vi "Main.vi"() -> ()   [LabVIEW 2026]
doc: "This LabVIEW application simulates scheduled programmatic heating and cooling control for heating, ventilation and air-conditioning (HVAC) system."
uses:
  controls/UI Data.ctl
  support/Message Queue/Enqueue Message (Single).vi
  <vilib>/Utility/error.llb/Error Cluster From Error Code.vi
  <vilib>/ErrorRing/Error Ring.xnode
  support/Message Queue/Message Queue.lvlib
  support/User Event - Stop/User Event - Stop.lvlib
  controls/Manual Override.ctl
  controls/System Status Displays.ctl
  controls/User Settings.ctl
panel:
  in  "User Settings":T1
  in  "Manual Override":T2
  out "System Status Displays":T3
  in  "Exit":bool
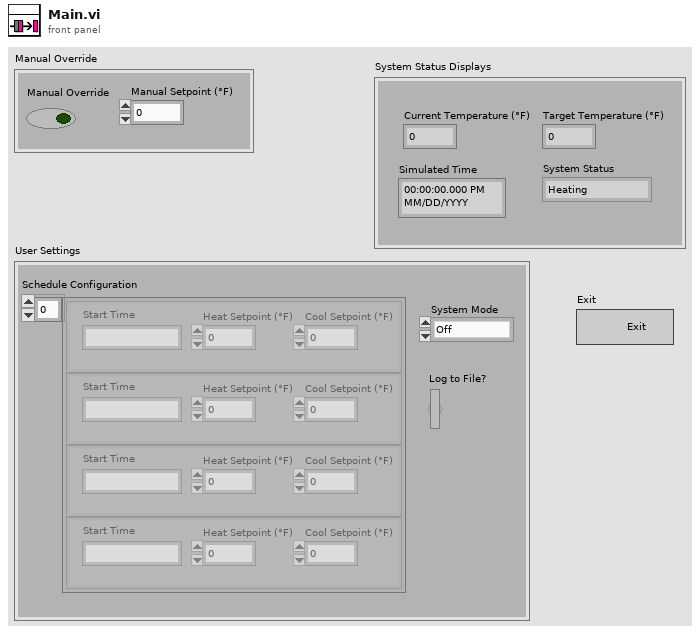
[diagram p1: front panel]
types:
  T1 = typedef "User Settings.ctl" = cluster{"Schedule Configuration":cluster{"Start Time":string, "Heat Setpoint (°F)":dbl, "Cool Setpoint (°F)":dbl}[], "System Mode":enum16{"Off", "Cool", "Auto", "Heat"}, "Log to File?":bool}
  T2 = typedef "Manual Override.ctl" = cluster{"Manual Override":bool, "Manual Setpoint (°F)":dbl}
  T3 = typedef "System Status Displays.ctl" = cluster{"Current Temperature (°F)":dbl, "Target Temperature (°F)":dbl, "System Status":enum16{"Heating", "Cooling", "Idle"}, "Simulated Time ":timestamp}
  T4 = typedef "UI Data.ctl" = cluster{"Boolean <Replace Me>":bool, "String <Replace Me>":string, "Numeric <Replace Me>":dbl, "Do Something Ref":refnum<vi>, "Do Something Else Ref":refnum<vi>, "Data Display Ref":refnum<vi>, "Exit Button Ref":refnum<vi>}
  T5 = typedef "Message Queue.lvlib/All Message Queues.ctl" = cluster{"UI":refnum<queue>}
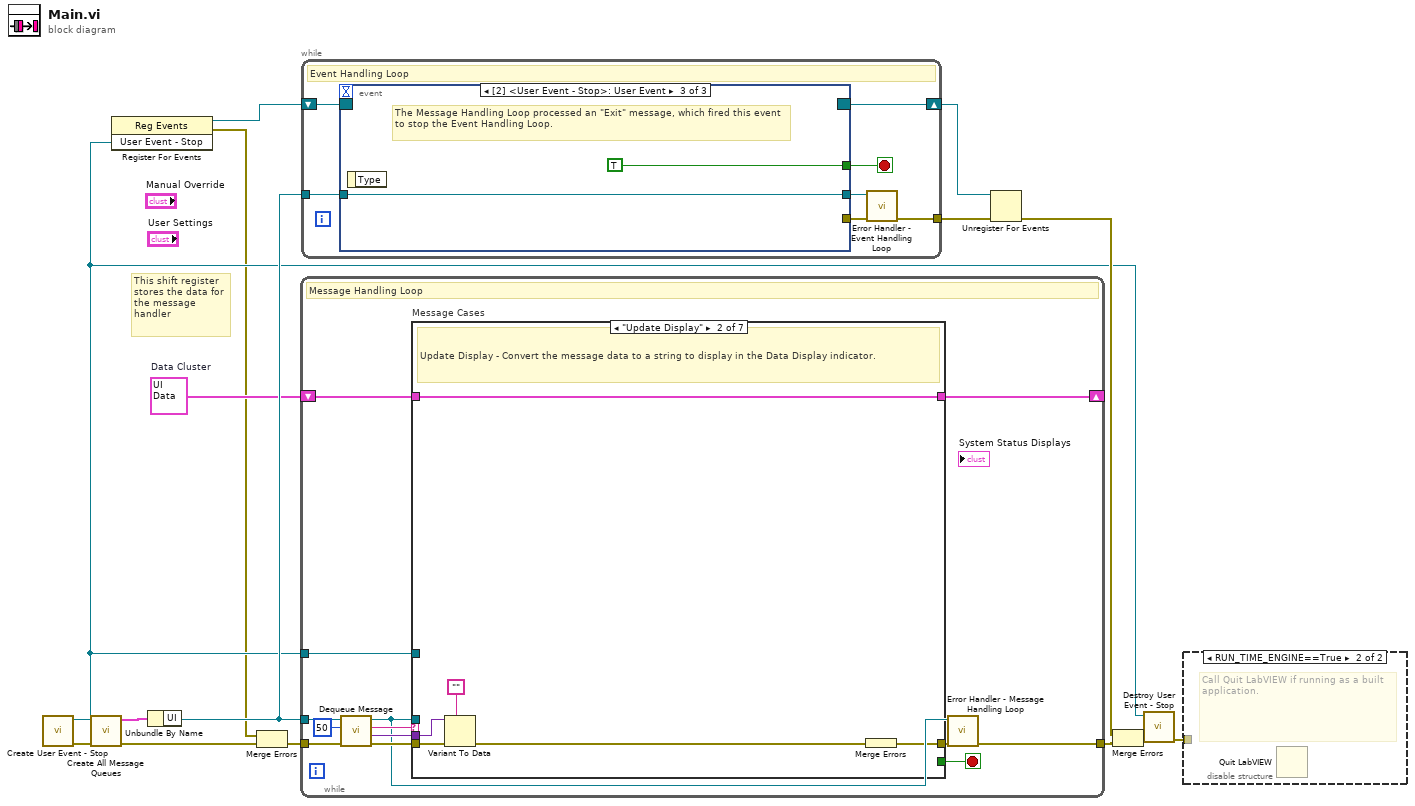
[diagram p0: block diagram]
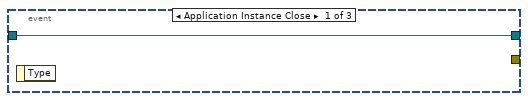
[diagram p3: hidden frame]
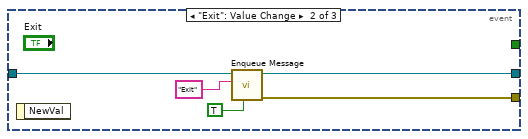
[diagram p4: hidden frame]
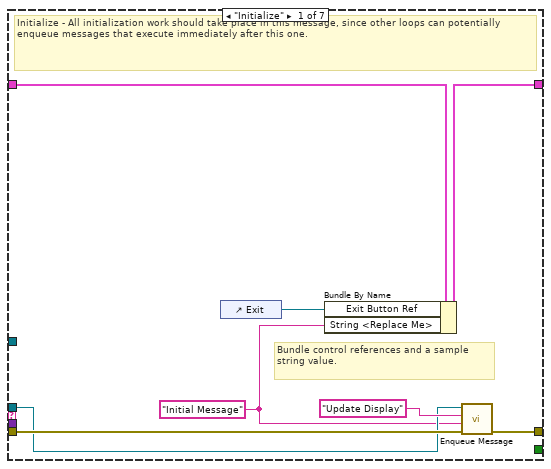
[diagram p5: hidden frame]
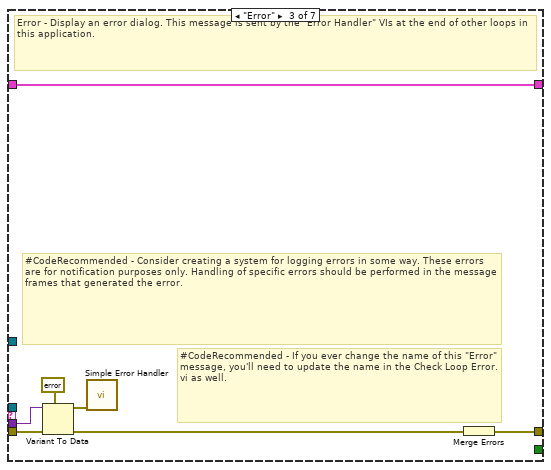
[diagram p6: hidden frame]
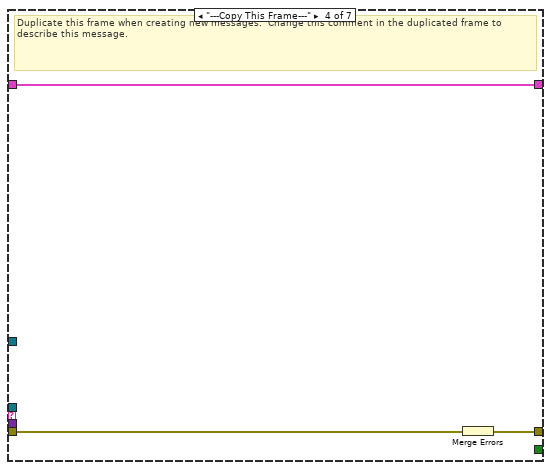
[diagram p7: hidden frame]
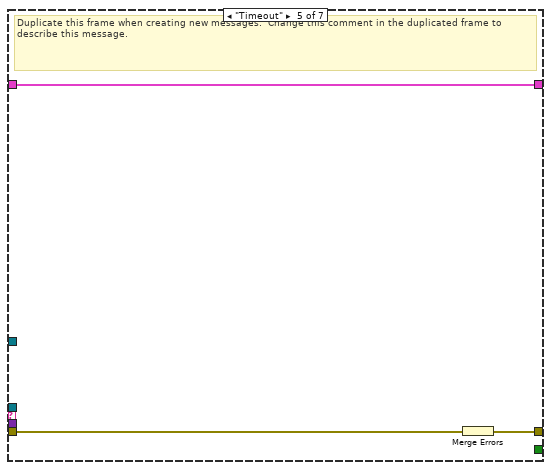
[diagram p8: hidden frame]
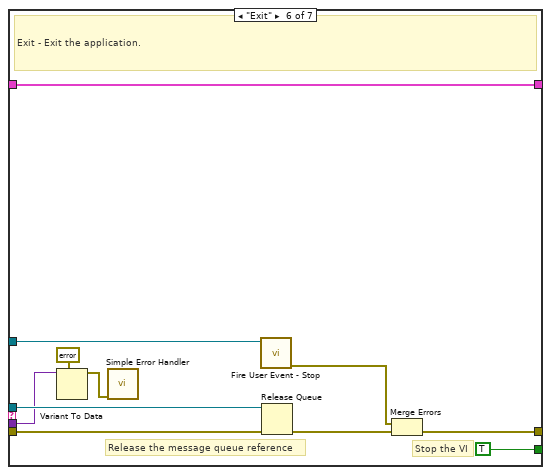
[diagram p9: hidden frame]
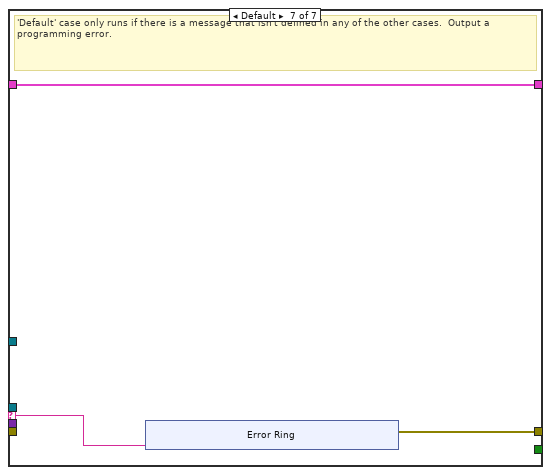
[diagram p10: hidden frame]
diagram:
  w7 = T4 {"Boolean <Replace Me>"=FALSE, "String <Replace Me>"="", "Numeric <Replace Me>"=0.0, "Do Something Ref"=refnum, "Do Something Else Ref"=refnum, "Data Display Ref"=refnum, "Exit Button Ref"=refnum}  # Data Cluster
  # "This shift register stores the data for the message handler"
  n1 = call "Create User Event - Stop.vi"() -> ("error out"=w11:errorcluster, "User Event - Stop"=w3:refnum<user-event>)  [unwired: 10 in]
  n2 = call "Create All Message Queues.vi"("error in (no error)"=w11) -> ("error out"=w15:errorcluster, "Message Queues out"=w14:T5)  [unwired: 9 in]
  n3 = register-events(w3) -> (reference out=w4:refnum<event-registration>, error out=w1:errorcluster)  [unwired: 2 in]
  n4 = Unbundle By Name(w14) -> ("UI"=w12:refnum<queue>)
  n5 = Merge Errors(w1, w15) -> (w2:errorcluster)
  n6 = while {
    tunnel: w12 -> [w20]
    shift-right: [w27] -> _
    shift-left: w7 -> [w28]
    tunnel: w3 -> [w25]
    tunnel: w2 -> [w24]
    tunnel: [w18] -> w13
    stop <- w26 stop-if-true
    # "Message Handling Loop"
    n7 = call "Dequeue Message.vi"("error in (no error)"=w24, "timeout in ms (-1)"=50, "Message Queue"=w20) -> ("error out"=w23:errorcluster, "Message Data"=w21:variant, "Message"=w22:string, "dup Message Queue"=w19:refnum<queue>)  [unwired: 5 in]
    n8 = case "Message Cases" shown="\"Update Display\"" w22 {
      selector: w22 -> [_ _ _ _ _ _ w67]
      tunnel: w19 -> [w30 _ _ _ _ w66 _]
      tunnel: w23 -> [w35 w40 w49 w52 w55 w59 _]
      tunnel: [w36 w41 w43 w50 w53 w62 w68] -> w17
      tunnel: w28 -> [w34 w42 w48 w51 w54 w65 w69]
      tunnel: [w33 w42 w48 w51 w54 w65 w69] -> w27
      tunnel: [_ _ _ _ _ TRUE _] -> w26
      tunnel: w21 -> [_ w39 w47 _ _ w56 _]
      tunnel: w25 -> [_ _ _ _ _ w61 _]
      frame "Initialize" {
        w29 = "Initial Message" ("Initial Message")
        # "Bundle control references and a sample string value."
        # "Initialize - All initialization work should take place in this message, since other loops can potentially enqueue messages that execute immediately after this one."
        n9 = control-ref of="Exit"() -> (w32:refnum<vi>)
        n10 = Bundle By Name(cluster=w34, "Exit Button Ref"=w32, "String <Replace Me>"=w29) -> (w33:T4)
        n11 = call-poly "Enqueue Message.vi"("error in (no error)"=w35, "Message Data"=w29, "Message"="Update Display", "Message Queue"=w30) -> ("error out"=w36:errorcluster)  [unwired: 6 in, 1 out]
      }
      frame "Update Display" {
        # "Update Display - Convert the message data to a string to display in the Data Display indicator."
        n12 = Variant To Data(error in=w40, type="", Variant=w39) -> (error out=w37:errorcluster)  [unwired: 1 out]
        n13 = Merge Errors(w37) -> (w41:errorcluster)
      }
      frame "Error" {
        # "#CodeRecommended - If you ever change the name of this \"Error\" message, you'll need to update the name in the Check Loop Error.vi as well."
        # "#CodeRecommended - Consider creating a system for logging errors in some way. These errors are for notification purposes only. Handling of specific errors should be performed in the message frames that generated the error."
        # "Error - Display an error dialog. This message is sent by the \"Error Handler\" VIs at the end of other loops in this application."
        n14 = Variant To Data(error in=w49, type=errorcluster {"status"=FALSE, "code"=0, "source"=""} ("error constant"), Variant=w47) -> (data=w45:errorcluster, error out=w44:errorcluster)
        n15 = call <vilib>:"Simple Error Handler.vi"("error in (no error)"=w45) -> ()  [unwired: 4 in, 5 out]
        n16 = Merge Errors(w44) -> (w43:errorcluster)
      }
      frame "---Copy This Frame---" {
        # "Duplicate this frame when creating new messages.  Change this comment in the duplicated frame to describe this message."
        n17 = Merge Errors(w52) -> (w50:errorcluster)
      }
      frame "Timeout" {
        # "Duplicate this frame when creating new messages.  Change this comment in the duplicated frame to describe this message."
        n18 = Merge Errors(w55) -> (w53:errorcluster)
      }
      frame "Exit" {
        # "Stop the VI"
        # "Release the message queue reference"
        # "Exit - Exit the application."
        n19 = Variant To Data(type=errorcluster {"status"=FALSE, "code"=0, "source"=""} ("error constant"), Variant=w56) -> (data=w57:errorcluster)  [unwired: 1 in, 1 out]
        n20 = call <vilib>:"Simple Error Handler.vi"("error in (no error)"=w57) -> ()  [unwired: 4 in, 5 out]
        n21 = call "Fire User Event - Stop.vi"("User Event - Stop"=w61) -> ("error out"=w60:errorcluster)  [unwired: 10 in]
        n22 = Release Queue(queue=w66, error in (no error)=w59) -> (error out=w63:errorcluster)  [unwired: 1 in, 2 out]
        n23 = Merge Errors(w60, w63) -> (w62:errorcluster)
      }
      frame Default {
        # "'Default' case only runs if there is a message that isn't defined in any of the other cases.  Output a programming error."
        n24 = xnode "Error Ring"("parameter 0"=w67) -> ("error out"=w68:errorcluster)
      }
    }
    n25 = call "Error Handler - Message Handling Loop.vi"("error in (no error)"=w17, "Message Queue"=w19) -> ("dup error in"=w18:errorcluster)  [unwired: 8 in, 1 out]
  }
  n26 = while {
    tunnel: w12 -> [w83]
    shift-right: [w81] -> w8
    shift-left: w4 -> [w82]
    tunnel: [w77] -> w5
    stop <- w79 stop-if-true
    # "Event Handling Loop"
    n27 = event shown="[2] <User Event - Stop>: User Event" {
      selector: w82 -> [_ _ _]
      dyn-events: [_ _ _] -> w81
      timeout: _ -> [_ _ _]
      tunnel: [_ _ TRUE ("Discard?")] -> w79
      tunnel: w83 -> [w84 w89 w91]
      tunnel: [_ w88 _] -> w80
      tunnel: [w84 w87 w91] -> w78
      event Application Instance Close {
        n28 = event-data() -> ()  [unwired: 1 in, 1 out]
      }
      event "Exit": Value Change {
        n29 = event-data() -> ()  [unwired: 1 in, 1 out]
        n30 = call-poly "Enqueue Message.vi"("Priority Message? (F)"=TRUE, "Message"="Exit", "Message Queue"=w89) -> ("error out"=w88:errorcluster, "dup Message Queue"=w87:refnum<queue>)  [unwired: 7 in]
      }
      event User Event {
        # "The Message Handling Loop processed an \"Exit\" message, which fired this event to stop the Event Handling Loop."
        n31 = event-data() -> ()  [unwired: 1 in, 1 out]
      }
    }
    n32 = call "Error Handler - Event Handling Loop.vi"("error in (no error)"=w80, "Message Queue"=w78) -> ("dup error in"=w77:errorcluster)  [unwired: 8 in, 1 out]
  }
  n33 = Unregister For Events(event registration refnum=w8, error in=w5) -> (error out=w9:errorcluster)
  n34 = Merge Errors(w9, w13) -> (w10:errorcluster)
  n35 = call "Destroy User Event - Stop.vi"("error in (no error)"=w10, "User Event - Stop"=w3) -> ("error out"=w6:errorcluster)  [unwired: 9 in]
  n36 = disable-structure shown="RUN_TIME_ENGINE==True" {
    disable-tunnel: w6 -> [_ _]
    frame condition #0 (active) {
    }
    frame condition #1 {
      # "Call Quit LabVIEW if running as a built application."
      n37 = Quit LabVIEW() -> ()  [unwired: 1 in]
    }
  }
